vi "Align & Distribute UI.vi"(6 "Predefined Input Key":string, 8 "error in (no error)":errorcluster, 9 "Panel Ref":refnum<vi>, 10 "Block Diagram Ref":refnum<vi>, 11 "Executed on Frontpanel?":bool) -> (0 "error out":errorcluster, 1 "Panel Ref out":refnum<vi>, 2 "Block Diagram Ref out":refnum<vi>)   [LabVIEW 2020, in "Align Elements.lvlib"]
uses:
  Align Elements.lvlib
  Align Objects.ctl
  Distribute Objects.ctl
  Dist Top Edges.ctl
  Dist Bottom Edges.ctl
  Dist Vertical Gap.ctl
  Dist Vertical Compress.ctl
  Dist Left Edges.ctl
  Dist Horizontal Centers.ctl
  Dist Right Edges.ctl
  Dist Horizontal Gap.ctl
  Dist Horizontal Compress.ctl
  <vilib>/Utility/inputDevices.llb/mouseAcquire.vi
  <vilib>/Utility/inputDevices.llb/closeMouse.vi
panel:
  in  "Distribute Objects":T1
  in  "Align Objects":T11
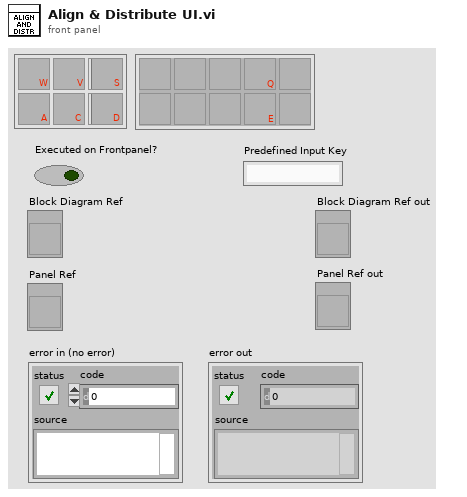
[diagram p1: front panel]
types:
  T1 = typedef "Align Elements.lvlib/Distribute Objects.ctl" = cluster{"Top Edges":T2, "Vertical Centers":bool, "Bottom Edges":T3, "Vertical Gap":T4, "Vertical Compress":T5, "Dist Left Edges":T6, "Dist Horizontal Centers":T7, "Dist Right Edges":T8, "Dist Horizontal Gap":T9, "Dist Horizontal Compress":T10}
  T2 = typedef "Align Elements.lvlib/Dist Top Edges.ctl" = bool
  T3 = typedef "Align Elements.lvlib/Dist Bottom Edges.ctl" = bool
  T4 = typedef "Align Elements.lvlib/Dist Vertical Gap.ctl" = bool
  T5 = typedef "Align Elements.lvlib/Dist Vertical Compress.ctl" = bool
  T6 = typedef "Align Elements.lvlib/Dist Left Edges.ctl" = bool
  T7 = typedef "Align Elements.lvlib/Dist Horizontal Centers.ctl" = bool
  T8 = typedef "Align Elements.lvlib/Dist Right Edges.ctl" = bool
  T9 = typedef "Align Elements.lvlib/Dist Horizontal Gap.ctl" = bool
  T10 = typedef "Align Elements.lvlib/Dist Horizontal Compress.ctl" = bool
  T11 = typedef "Align Elements.lvlib/Align Objects.ctl" = cluster{"Top Edges":bool, "Vertical Centers":bool, "Bottom Edges":bool, "Left Edges":bool, "Horizontal Centers":bool, "Right Edges":bool}
  T12 = cluster{"Horizontal":i32, "Vertical":i32, "Scrolling":i32}
  T13 = enum32{"Invalid", "Standard", "Closed", "Hidden", "Minimized", "Maximized"}
  T14 = enum32{"Top Edges", "Vertical Centers", "Bottom Edges", "Left Edges", "Horizontal Centers", "Right Edges"}
  T15 = enum32{"Top Edges", "Vertical Centers", "Bottom Edges", "Vertical Gap", "Vertical Compress", "Left Edges", "Horizontal Centers", "Right Edges", "Horizontal Gap", "Horizontal Compress"}
  T16 = typedef "eventvkey.ctl" = enum16{"ASCII", "Enter", "Return", "Shift", "Ctrl", "Alt", "Cmd", "Opt", "Caps", "NumLock", "Clear", "Break", "Up", "Down", "Left", "Right", "Insert", "Delete", "Home", "End", "PageUp", "PageDown", "Escape", "Help", "Pause", "ScrollLock", "F1", "F2", "F3", "F4", "F5", "F6", "F7", "F8", "F9", "F10", "F11", "F12", "F13", "F14", "F15", "F16", "F17", "F18", "F19", "F20", "F21", "F22", "F23", "F24", "Play", "VolumeUp", "VolumeDown", "Mute", "Two Byte Char"}
  T17 = typedef "LVRectTypeDef.ctl" = cluster{"Left":i16, "Top":i16, "Right":i16, "Bottom":i16}
  T18 = cluster{"Horizontal":i16, "Vertical":i16, "Scrolling":i16}
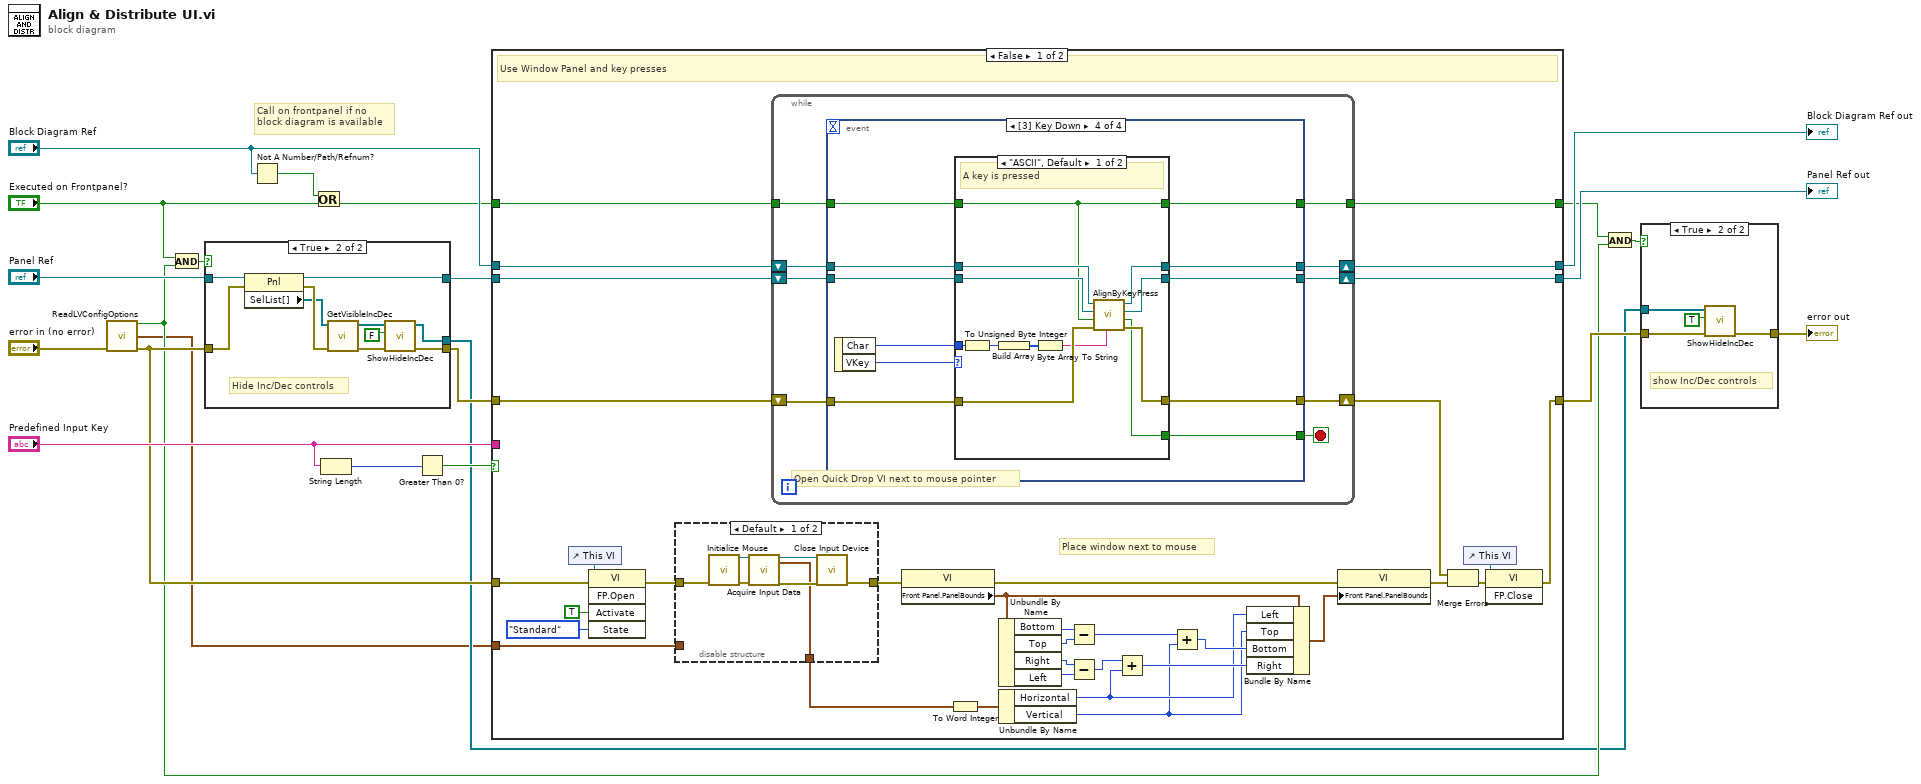
[diagram p0: block diagram]
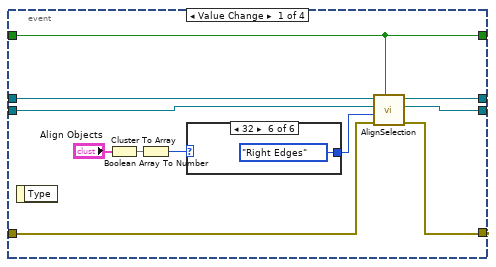
[diagram p3: hidden frame]
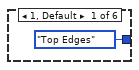
[diagram p4: hidden frame]
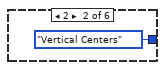
[diagram p5: hidden frame]
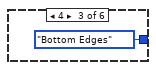
[diagram p6: hidden frame]
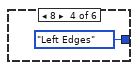
[diagram p7: hidden frame]
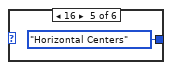
[diagram p8: hidden frame]
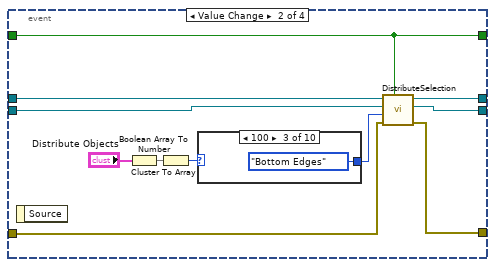
[diagram p9: hidden frame]
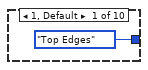
[diagram p10: hidden frame]
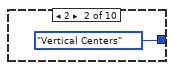
[diagram p11: hidden frame]
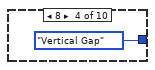
[diagram p12: hidden frame]
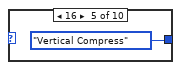
[diagram p13: hidden frame]
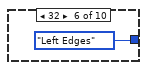
[diagram p14: hidden frame]
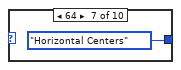
[diagram p15: hidden frame]
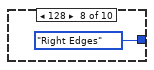
[diagram p16: hidden frame]
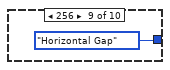
[diagram p17: hidden frame]
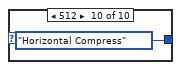
[diagram p18: hidden frame]
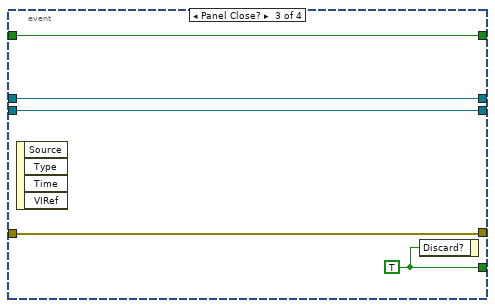
[diagram p19: hidden frame]
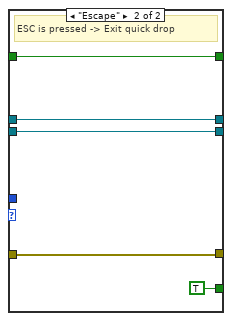
[diagram p20: hidden frame]
diagram:
  # "Call on frontpanel if no\nblock diagram is available"
  n1 = call "ReadLVConfigOptions.vi"("error in"="error in (no error)") -> ("HideIncDec?"=w6:bool, "WinPosOffset"=w1:T12, "error out"=w9:errorcluster)  [unwired: 12 in]
  n2 = And(x="Executed on Frontpanel?", y=w6) -> (x .and. y?=w10:bool)
  n3 = case shown="True" w10 {
    tunnel: [_ w26] -> w5
    tunnel: [w23 w28] -> w18
    tunnel: "Panel Ref" -> [w24 w32]
    tunnel: [w24 w31] -> w19
    tunnel: w9 -> [w23 w30]
    frame False {
    }
    frame True {
      # "Hide Inc/Dec controls"
      n4 = property class="Pnl"(reference=w32, error in=w30) -> (reference out=w31:refnum<vi>, error out=w34:errorcluster, "SelList[]"=w29:refnum<vi>[])
      n5 = call "GetVisibleIncDec.vi"("error in"=w34, "SelList[]"=w29) -> ("error out"=w33:errorcluster, "NumericRefs"=w27:refnum<vi>[])  [unwired: 8 in]
      n6 = call "ShowHideIncDec.vi"("error in (no error)"=w33, "Show?"=FALSE, "NumericRefs"=w27) -> ("error out"=w28:errorcluster, "NumericRefs out"=w26:refnum<vi>[])  [unwired: 7 in]
    }
  }
  n7 = Not A Number/Path/Refnum?(number/path/refnum="Block Diagram Ref") -> (NaN/Path/Refnum?=w2:bool)
  n8 = Or(x=w2, y="Executed on Frontpanel?") -> (x .or. y?=w3:bool)
  n9 = String Length(string="Predefined Input Key") -> (length=w21:i32)
  n10 = Greater Than 0?(x=w21) -> (x > 0?=w20:bool)
  n11 = case shown="False" w20 {
    tunnel: w9 -> [w51 _]
    tunnel: "Block Diagram Ref" -> [w47 w163]
    tunnel: w19 -> [w46 w164]
    tunnel: w18 -> [w45 w161]
    tunnel: w3 -> [w44 w160]
    tunnel: [w43 w165] -> w17
    tunnel: [w42 w166] -> w16
    tunnel: [w39 w162] -> w15
    tunnel: [w41 w160] -> w14
    tunnel: "Predefined Input Key" -> [_ w159]
    tunnel: w1 -> [w35 _]
    frame False {
      # "Place window next to mouse"
      # "Open Quick Drop VI next to mouse pointer"
      # "Use Window Panel and key presses"
      n12 = control-ref of="This VI"() -> (w52:refnum<vi>)
      n13 = invoke class="VI" method="FP.Open"(reference=w52, error in=w51, "Activate"=TRUE ("Activate?"), "State"=T13."Standard") -> (error out=w50:errorcluster)  [unwired: 1 in, 4 out]
      n14 = disable-structure shown="Default" {
        disable-tunnel: [w71 w76] -> w68
        disable-tunnel: [w70 w77] -> w57
        disable-tunnel: w50 -> [w69 w77]
        disable-tunnel: w35 -> [_ w76]
        frame condition #0 (active) {
          n15 = call <vilib>:"Initialize Mouse.vi"("error in (no error)"=w69) -> ("error out"=w75:errorcluster, "device ID"=w74:refnum<k1>)  [unwired: 9 in]
          n16 = call-poly <vilib>:"Acquire Input Data.vi"("device ID"=w74, "error in (no error)"=w75) -> ("device ID"=w72:refnum<k1>, "axis info"=w71:T12, "error out"=w73:errorcluster)  [unwired: 14 in, 1 out]
          n17 = call-poly <vilib>:"Close Input Device.vi"("error in (no error)"=w73, "device ID"=w72) -> ("error out"=w70:errorcluster)  [unwired: 8 in]
        }
        frame condition #1 {
        }
      }
      n18 = while {
        shift-right: [w86] -> w43
        shift-left: w47 -> [w85]
        shift-right: [w84] -> w42
        shift-left: w46 -> [w83]
        shift-right: [w82] -> w37
        shift-left: w45 -> [w81]
        tunnel: [w80] -> w41
        tunnel: w44 -> [w79]
        stop <- w78 stop-if-true
        n19 = event shown="[3] Key Down" {
          selector: _ -> [_ _ _ _]
          dyn-events: _ -> [_ _ _ _]
          timeout: _ -> [_ _ _ _]
          tunnel: [w91 w109 w128 w138] -> w86
          tunnel: w85 -> [w93 w111 w128 w139]
          tunnel: [w90 w108 w127 w136] -> w84
          tunnel: w83 -> [w92 w110 w127 w137]
          tunnel: [w87 w107 w125 w133] -> w82
          tunnel: w81 -> [w88 w106 w125 w134]
          tunnel: [w94 w105 w129 w131] -> w80
          tunnel: w79 -> [w94 w105 w129 w135]
          tunnel: [_ _ w126 w130] -> w78
          event Value Change {
            n20 = event-data() -> ()  [unwired: 1 in, 1 out]
            n21 = Cluster To Array(cluster="Align Objects") -> (array=w96:bool[])
            n22 = Boolean Array To Number(Boolean array=w96) -> (number=w95:u32)
            n23 = case shown="32" w95 {
              tunnel: [T14."Top Edges" ("Align Type") T14."Vertical Centers" ("Align Type") T14."Bottom Edges" ("Align Type") T14."Left Edges" ("Align Type") T14."Horizontal Centers" ("Align Type") T14."Right Edges" ("Align Type")] -> w89
              frame 1, Default {
              }
              frame 2 {
              }
              frame 4 {
              }
              frame 8 {
              }
              frame 16 {
              }
              frame 32 {
              }
            }
            n24 = call "AlignSelection.vi"("Executed on Frontpanel?"=w94, "error in (no error)"=w88, "Align Type"=w89, "Panel Ref in"=w92, "TopLevelDiagram in"=w93) -> ("error out"=w87:errorcluster, "Panel Ref out"=w90:refnum<vi>, "TopLevelDiagram out"=w91:refnum<vi>)  [unwired: 4 in]
          }
          event Value Change {
            n25 = event-data() -> ()  [unwired: 1 in, 1 out]
            n26 = Cluster To Array(cluster="Distribute Objects") -> (array=w114:T10[])
            n27 = Boolean Array To Number(Boolean array=w114) -> (number=w113:u32)
            n28 = case shown="100" w113 {
              tunnel: [T15."Top Edges" ("DistributeType") T15."Vertical Centers" ("DistributeType") T15."Bottom Edges" ("DistributeType") T15."Vertical Gap" ("DistributeType") T15."Vertical Compress" ("DistributeType") T15."Left Edges" ("DistributeType") T15."Horizontal Centers" ("DistributeType") T15."Right Edges" ("DistributeType") T15."Horizontal Gap" ("DistributeType") T15."Horizontal Compress" ("DistributeType")] -> w104
              frame 1, Default {
              }
              frame 2 {
              }
              frame 4 {
              }
              frame 8 {
              }
              frame 16 {
              }
              frame 32 {
              }
              frame 64 {
              }
              frame 128 {
              }
              frame 256 {
              }
              frame 512 {
              }
            }
            n29 = call "DistributeSelection.vi"("Executed on Frontpanel?"=w105, "error in (no error)"=w106, "DistributeType"=w104, "Panel Ref in"=w110, "TopLevelDiagram in"=w111) -> ("error out"=w107:errorcluster, "Panel Ref out"=w108:refnum<vi>, "TopLevelDiagram out"=w109:refnum<vi>)  [unwired: 4 in]
          }
          event Panel Close? {
            w126 = TRUE
            n30 = event-data() -> ()  [unwired: 1 in, 4 out]
            n31 = event-data("Discard?"=w126) -> ()  [unwired: 1 in, 1 out]
          }
          event Key Down {
            n32 = event-data() -> ("Char"=w140:i16, "VKey"=w132:T16)  [unwired: 1 in]
            n33 = case shown="\"ASCII\", Default" w132 {
              tunnel: w140 -> [w150 _]
              tunnel: w139 -> [w149 w156]
              tunnel: [w148 w156] -> w138
              tunnel: w137 -> [w147 w155]
              tunnel: [w146 w155] -> w136
              tunnel: w135 -> [w142 w157]
              tunnel: w134 -> [w145 w154]
              tunnel: [w144 w154] -> w133
              tunnel: [w142 w157] -> w131
              tunnel: [w143 TRUE] -> w130
              frame "ASCII", Default {
                # "A key is pressed"
                n34 = To Unsigned Byte Integer(number=w150) -> (unsigned 8bit integer=w151:u8)
                n35 = Build Array(w151) -> (w152:u8[])
                n36 = Byte Array To String(unsigned byte array=w152) -> (string=w141:string)
                n37 = call "AlignByKeyPress.vi"("KeyChar"=w141, "error in (no error)"=w145, "Executed on Frontpanel?"=w142, "Panel Ref"=w147, "TopLevelDiagram in"=w149) -> ("error out"=w144:errorcluster, "Align Executed?"=w143:bool, "Panel Ref out"=w146:refnum<vi>, "TopLevelDiagram out"=w148:refnum<vi>)  [unwired: 3 in]
              }
              frame "Escape" {
                # "ESC is pressed -> Exit quick drop"
              }
            }
          }
        }
      }
      n38 = property class="VI"(error in=w57) -> (error out=w58:errorcluster, "Front Panel.PanelBounds"=w66:T17)  [unwired: 1 in, 1 out]
      n39 = To Word Integer(number=w68) -> (16bit integer=w61:T18)
      n40 = Unbundle By Name(w66) -> ("Bottom"=w65:i16, "Top"=w64:i16, "Right"=w63:i16, "Left"=w62:i16)
      n41 = Unbundle By Name(w61) -> ("Horizontal"=w54:i16, "Vertical"=w53:i16)
      n42 = Subtract(x=w65, y=w64) -> (x-y=w56:i16)
      n43 = Subtract(x=w63, y=w62) -> (x-y=w55:i16)
      n44 = Add(x=w55, y=w54) -> (x+y=w59:i16)
      n45 = Add(x=w56, y=w53) -> (x+y=w60:i16)
      n46 = Bundle By Name(cluster=w66, "Left"=w54, "Top"=w53, "Bottom"=w60, "Right"=w59) -> (w67:T17)
      n47 = property class="VI"(error in=w58, "Front Panel.PanelBounds"=w67) -> (error out=w36:errorcluster)  [unwired: 1 in, 1 out]
      n48 = Merge Errors(w37, w36) -> (w38:errorcluster)
      n49 = control-ref of="This VI"() -> (w40:refnum<vi>)
      n50 = invoke class="VI" method="FP.Close"(reference=w40, error in=w38) -> (error out=w39:errorcluster)  [unwired: 1 in, 2 out]
    }
    frame True {
      # "Use string from quickdrop combo box."
      n51 = String To Byte Array(string=w159) -> (unsigned byte array=w158:u8[])
      n52 = for {
        tunnel: w160 -> [w169]
        tunnel: w158 -> [w168] mode=indexing
        shift-right: [w175] -> w166
        shift-left: w164 -> [w173]
        shift-right: [w174] -> w165
        shift-left: w163 -> [w172]
        shift-right: [w171] -> w162
        shift-left: w161 -> [w170]
        n53 = Type Cast(x=w168) -> (*(type *) &x=w167:string)  [unwired: 1 in]
        n54 = call "AlignByKeyPress.vi"("KeyChar"=w167, "error in (no error)"=w170, "Executed on Frontpanel?"=w169, "Panel Ref"=w173, "TopLevelDiagram in"=w172) -> ("error out"=w171:errorcluster, "Panel Ref out"=w175:refnum<vi>, "TopLevelDiagram out"=w174:refnum<vi>)  [unwired: 3 in, 1 out]
      }
    }
  }
  "Block Diagram Ref out" <- w17
  "Panel Ref out" <- w16
  n55 = And(x=w14, y=w6) -> (x .and. y?=w7:bool)
  n56 = case shown="True" w7 {
    tunnel: w5 -> [_ w178]
    tunnel: w15 -> [w176 w179]
    tunnel: [w176 w177] -> w13
    frame False {
    }
    frame True {
      # "show Inc/Dec controls"
      n57 = call "ShowHideIncDec.vi"("error in (no error)"=w179, "Show?"=TRUE, "NumericRefs"=w178) -> ("error out"=w177:errorcluster)  [unwired: 7 in, 1 out]
    }
  }
  "error out" <- w13
